vi "Calculate Temperature.vi"(4 "Temperature Data":string="ThermBias=1780 ThermInput=1393 ThermOffset=584") -> (1 "Temperature":dbl)   [LabVIEW 2010]
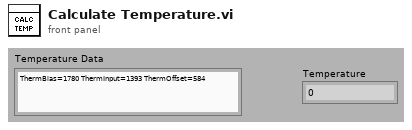
[diagram p1: front panel]
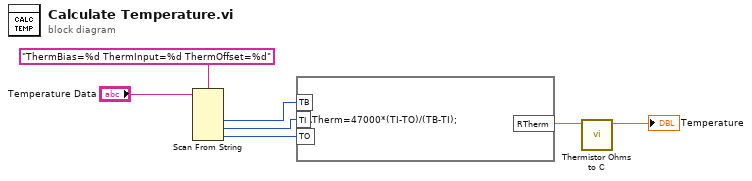
[diagram p0: block diagram]
diagram:
  n1 = Scan From String(format string="ThermBias=%d ThermInput=%d ThermOffset=%d", input string="Temperature Data") -> (output 1=w5:i32, output 2=w4:i32, output 3=w3:i32)  [unwired: 5 in, 3 out]
  n2 = formula code="RTherm=47000*(TI-TO)/(TB-TI);"("TB"=w5, "TI"=w4, "TO"=w3) -> ("RTherm"=w2:dbl)
  n3 = call "Thermistor Ohms to C.vi"("Thermistor R"=w2) -> ("Thermistor C"=→"Temperature":dbl)  [unwired: 10 in]
